vi "InterpretCLI.vi"(11 "Path":path) -> (1 "Strings":string[](array[string]), 2 "Layers":i32, 3 "Commands":T1(array[cluster]))   [LabVIEW 2012]
panel:
  out "MissedCommands":u16[](array[numeric])
  out "Command":u16
  out "TotalSize":i32
  out "Command":string
  out "Data":string
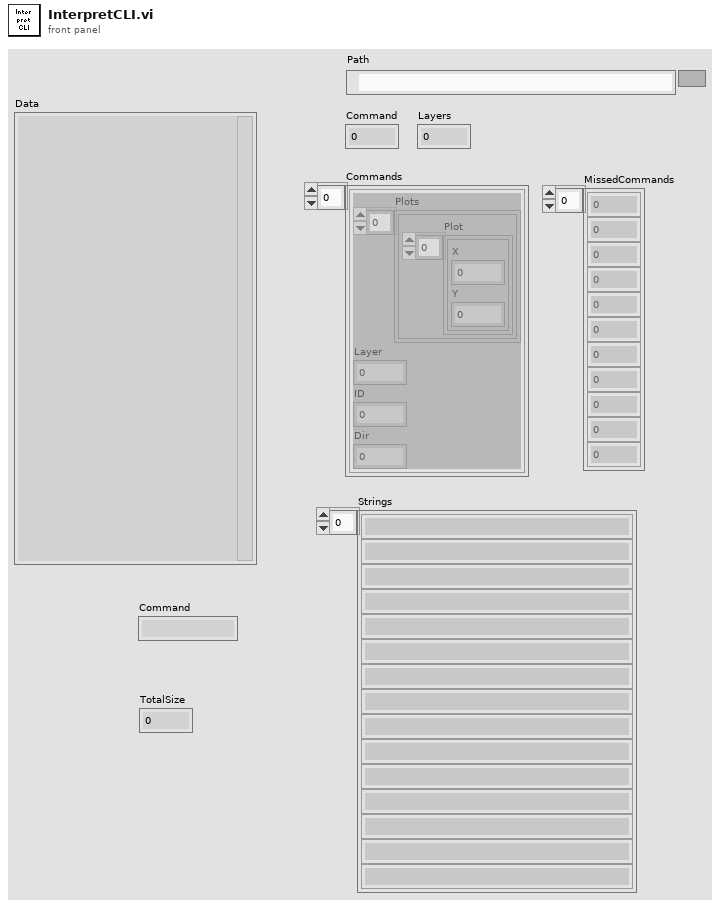
[diagram p1: front panel]
types:
  T1 = cluster{"Plots":cluster{"Plot":cluster{"X":dbl, "Y":dbl}[]}[], "Layer":dbl, "ID":dbl, "Dir":dbl}[]
  T2 = cluster{"Plots":cluster{"Plot":cluster{"X":dbl, "Y":dbl}[]}[], "Layer":dbl, "ID":dbl, "Dir":dbl}
  T3 = enum16{"big-endian, network order", "native, host order", "little-endian"}
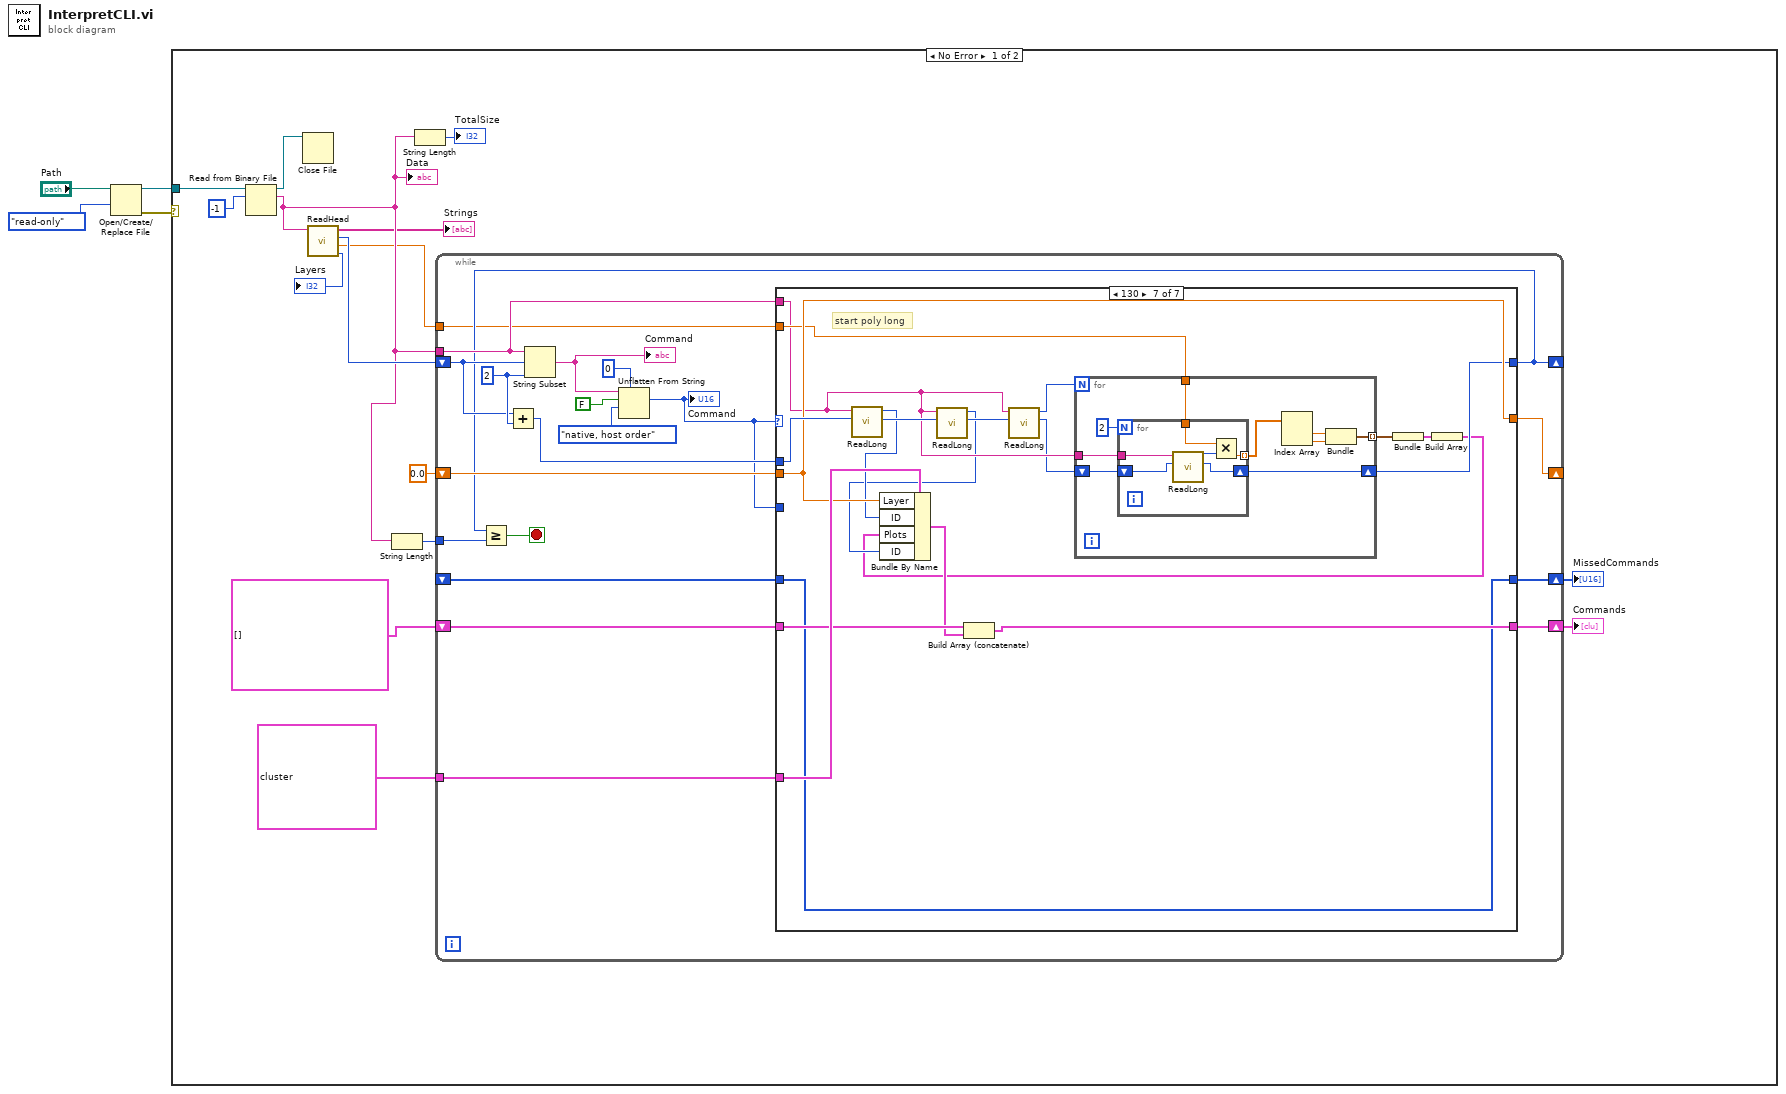
[diagram p0: block diagram]
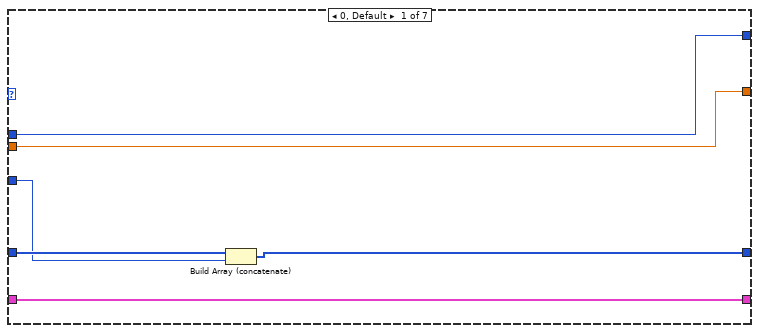
[diagram p2: hidden frame]
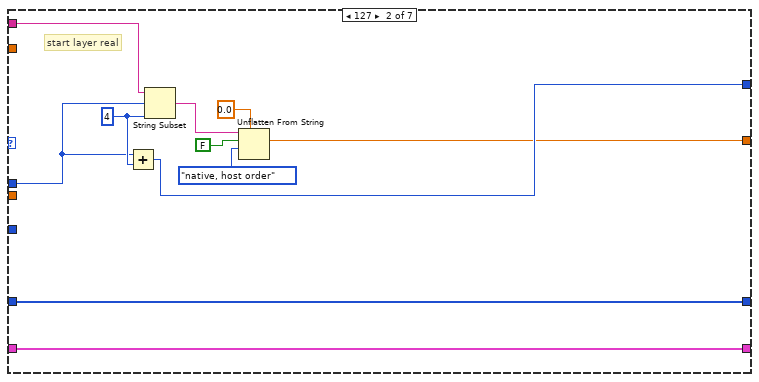
[diagram p3: hidden frame]
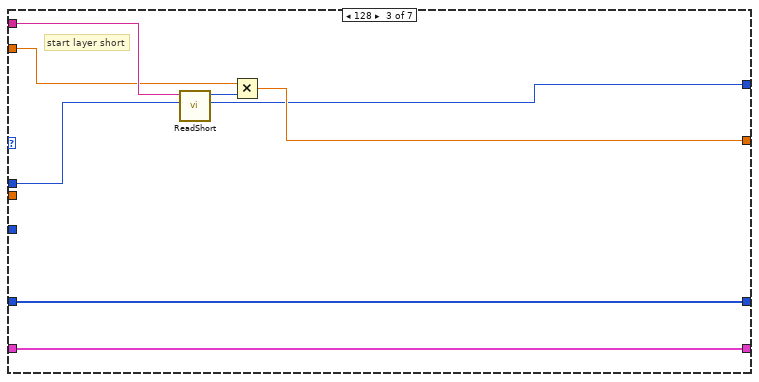
[diagram p4: hidden frame]
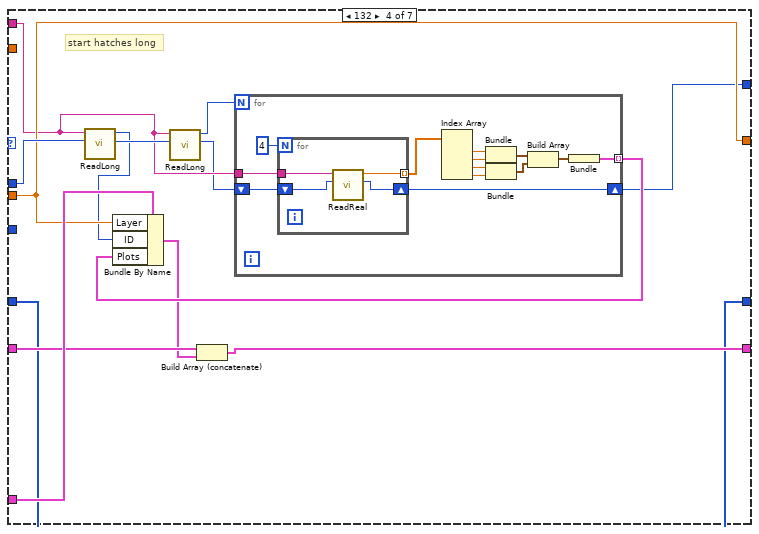
[diagram p5: hidden frame]
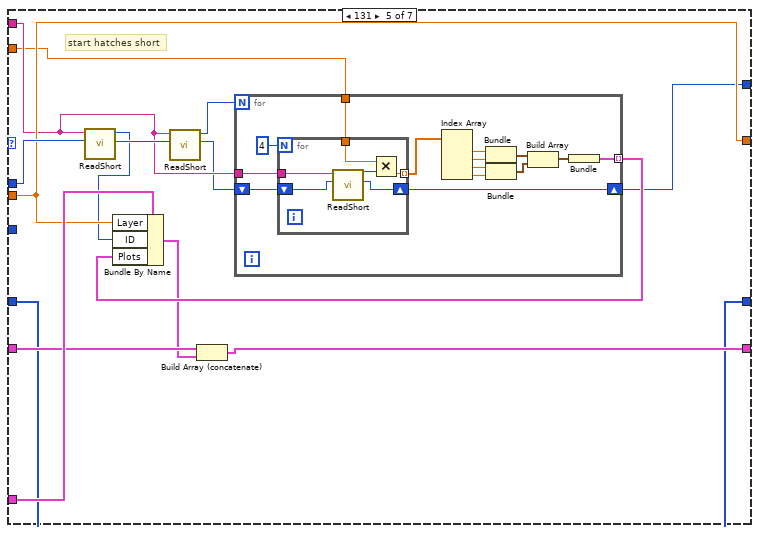
[diagram p6: hidden frame]
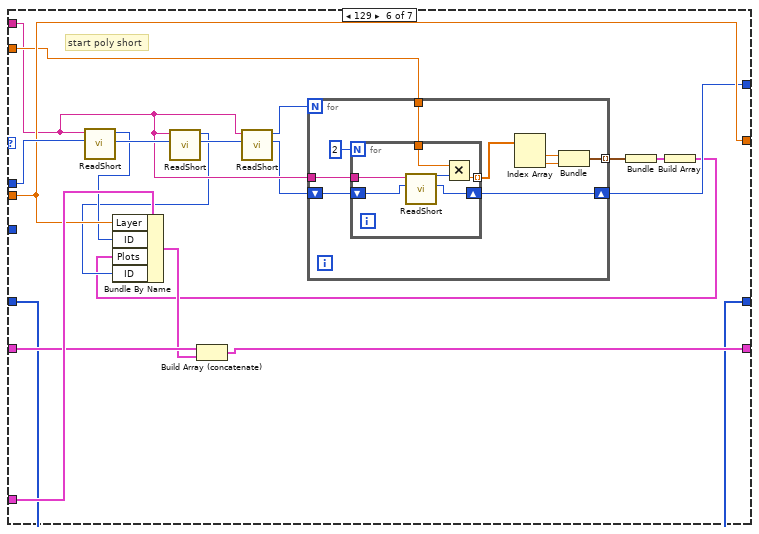
[diagram p7: hidden frame]
diagram:
  n1 = Open/Create/Replace File(file path (use dialog)="Path", access (0:read/write)=enum16{"read/write", "read-only", "write-only"}."read-only") -> (refnum out=w3:refnum<file>, error out=w1:errorcluster)  [unwired: 4 in, 1 out]
  n2 = case shown="No Error" w1 {
    tunnel: w3 -> [w19 _]
    frame No Error {
      n3 = Read from Binary File(10:-1 ("count (1)"), 11:w19) -> (2:w14:string, 3:w17:refnum<file>)  [unwired: 4 in, 2 out]
      "Data" <- w14
      n4 = Close File(refnum=w17) -> ()  [unwired: 1 in, 2 out]
      n5 = call "ReadHead.vi"("Data"=w14) -> ("Layers"=→"Layers":i32, "Units"=w6:dbl, "Off"=w15:u32, "Strings"=→"Strings":string[])  [unwired: 7 in]
      n6 = String Length(string=w14) -> (length=w12:i32)
      n7 = String Length(string=w14) -> (length=→"TotalSize":i32)
      n8 = while {
        tunnel: w14 -> [w33]
        shift-right: [w28] -> _
        shift-left: w15 -> [w29]
        shift-right: [w32] -> _
        shift-left: sgl 0.0 ("length (rest)") -> [w31]
        tunnel: w12 -> [w27]
        shift-right: [w25] -> w9
        shift-left: T1 [] -> [w24]
        tunnel: T2 {"Plots"=[{"Plot"=[{"X"=0.0, "Y"=0.0}, {"X"=1.0, "Y"=1.0}]}, {"Plot"=[{"X"=0.0, "Y"=1.0}, {"X"=1.0, "Y"=0.0}]}], "Layer"=0.0, "ID"=0.0, "Dir"=0.0} ("Command") -> [w26]
        shift-right: [w21] -> w7
        shift-left: _ -> [w22]
        tunnel: w6 -> [w20]
        stop <- w30 stop-if-true
        w35 = 2 ("length (rest)")
        n9 = Add(x=w29, y=w35) -> (x+y=w34:u32)
        n10 = String Subset(string=w33, offset (0)=w29, length (rest)=w35) -> (substring=w37:string)
        "Command" <- w37
        n11 = Unflatten From String(type=u16 0 ("length (rest)"), binary string=w37, data includes array or string size? (T)=FALSE, byte order (0:big-endian, network order)=T3."native, host order") -> (value=w23:u16)  [unwired: 1 in, 2 out]
        "Command" <- w23
        n12 = case shown="130" w23 {
          tunnel: w34 -> [w44 w50 w61 w78 w110 w149 w183]
          tunnel: w33 -> [_ w51 w62 w72 w104 w138 w172]
          tunnel: [w44 w49 w57 w69 w101 w144 w178] -> w28
          tunnel: [w45 w48 w58 w75 w107 w146 w180] -> w32
          tunnel: w31 -> [w45 _ _ w75 w107 w146 w180]
          tunnel: w26 -> [_ _ _ w76 w108 w147 w181]
          tunnel: [w43 w47 w64 w66 w98 w141 w175] -> w25
          tunnel: w24 -> [w43 w47 w64 w68 w100 w143 w177]
          tunnel: w23 -> [w41 _ _ _ _ _ _]
          tunnel: w22 -> [w42 w46 w63 w65 w97 w140 w174]
          tunnel: [w40 w46 w63 w65 w97 w140 w174] -> w21
          tunnel: w20 -> [_ _ w59 _ w96 w139 w173]
          frame 0, Default {
            n13 = Build Array (concatenate)(w42, w41) -> (w40:u16[])
          }
          frame 127 {
            w56 = 4 ("length (rest)")
            # "start layer real"
            n14 = Add(x=w50, y=w56) -> (x+y=w49:u32)
            n15 = String Subset(string=w51, offset (0)=w50, length (rest)=w56) -> (substring=w54:string)
            n16 = Unflatten From String(type=sgl 0.0 ("length (rest)"), binary string=w54, data includes array or string size? (T)=FALSE, byte order (0:big-endian, network order)=T3."native, host order") -> (value=w48:sgl)  [unwired: 1 in, 2 out]
          }
          frame 128 {
            # "start layer short"
            n17 = call "ReadShort.vi"("Offset"=w61, "Data"=w62) -> ("OffsetOut"=w57:u32, "Value"=w60:u16)  [unwired: 8 in]
            n18 = Multiply(x=w59, y=w60) -> (x*y=w58:dbl)
          }
          frame 132 {
            # "start hatches long"
            n19 = call "ReadLong.vi"("Offset"=w78, "Data"=w72) -> ("OffsetOut"=w77:u32, "Value"=w74:u32)  [unwired: 8 in]
            n20 = call "ReadLong.vi"("Offset"=w77, "Data"=w72) -> ("OffsetOut"=w71:u32, "Value"=w73:u32)  [unwired: 8 in]
            n21 = for {
              N: w73 -> [_]
              tunnel: w72 -> [w91]
              shift-right: [w88] -> w69
              shift-left: w71 -> [w89]
              tunnel: [w79] -> w70 mode=indexing
              n22 = for {
                N: 4 -> [_]
                tunnel: w91 -> [w95]
                shift-right: [w93] -> w88
                shift-left: w89 -> [w94]
                tunnel: [w92] -> w87 mode=indexing
                n23 = call "ReadReal.vi"("Offset"=w94, "Data"=w95) -> ("OffsetOut"=w93:u32, "Value"=w92:sgl)  [unwired: 8 in]
              }
              n24 = Index Array(array=w87) -> (element #1=w86:sgl, element #2=w85:sgl, element #3=w84:sgl, element #4=w83:sgl)  [unwired: 4 in]
              n25 = Bundle("Value"=w86, "Value"=w85) -> (w82:cluster{"Value":sgl, "Value":sgl})  [unwired: 1 in]
              n26 = Bundle("Value"=w84, "Value"=w83) -> (w81:cluster{"Value":sgl, "Value":sgl})  [unwired: 1 in]
              n27 = Build Array(w82, w81) -> (w80:cluster{"Value":sgl, "Value":sgl}[])
              n28 = Bundle(w80) -> (w79:cluster{cluster{"Value":sgl, "Value":sgl}[]})  [unwired: 1 in]
            }
            n29 = Bundle By Name(cluster=w76, "Layer"=w75, "ID"=w74, "Plots"=w70) -> (w67:T2)
            n30 = Build Array (concatenate)(w68, w67) -> (w66:T1)
          }
          frame 131 {
            # "start hatches short"
            n31 = call "ReadShort.vi"("Offset"=w110, "Data"=w104) -> ("OffsetOut"=w109:u32, "Value"=w106:u16)  [unwired: 8 in]
            n32 = call "ReadShort.vi"("Offset"=w109, "Data"=w104) -> ("OffsetOut"=w103:u32, "Value"=w105:u16)  [unwired: 8 in]
            n33 = for {
              N: w105 -> [_]
              tunnel: w104 -> [w124]
              shift-right: [w121] -> w101
              shift-left: w103 -> [w122]
              tunnel: [w112] -> w102 mode=indexing
              tunnel: w96 -> [w111]
              n34 = for {
                N: 4 -> [_]
                tunnel: w124 -> [w130]
                shift-right: [w128] -> w121
                shift-left: w122 -> [w129]
                tunnel: [w126] -> w120 mode=indexing
                tunnel: w111 -> [w125]
                n35 = call "ReadShort.vi"("Offset"=w129, "Data"=w130) -> ("OffsetOut"=w128:u32, "Value"=w127:u16)  [unwired: 8 in]
                n36 = Multiply(x=w125, y=w127) -> (x*y=w126:dbl)
              }
              n37 = Index Array(array=w120) -> (element #1=w119:dbl, element #2=w118:dbl, element #3=w117:dbl, element #4=w116:dbl)  [unwired: 4 in]
              n38 = Bundle(w119, w118) -> (w115:cluster{dbl, dbl})  [unwired: 1 in]
              n39 = Bundle(w117, w116) -> (w114:cluster{dbl, dbl})  [unwired: 1 in]
              n40 = Build Array(w115, w114) -> (w113:cluster{dbl, dbl}[])
              n41 = Bundle(w113) -> (w112:cluster{cluster{dbl, dbl}[]})  [unwired: 1 in]
            }
            n42 = Bundle By Name(cluster=w108, "Layer"=w107, "ID"=w106, "Plots"=w102) -> (w99:T2)
            n43 = Build Array (concatenate)(w100, w99) -> (w98:T1)
          }
          frame 129 {
            # "start poly short"
            n44 = call "ReadShort.vi"("Offset"=w149, "Data"=w138) -> ("OffsetOut"=w148:u32, "Value"=w145:u16)  [unwired: 8 in]
            n45 = call "ReadShort.vi"("Offset"=w148, "Data"=w138) -> ("OffsetOut"=w137:u32, "Value"=w134:u16)  [unwired: 8 in]
            n46 = call "ReadShort.vi"("Offset"=w137, "Data"=w138) -> ("OffsetOut"=w136:u32, "Value"=w135:u16)  [unwired: 8 in]
            n47 = for {
              N: w135 -> [_]
              tunnel: w138 -> [w158]
              shift-right: [w155] -> w144
              shift-left: w136 -> [w156]
              tunnel: [w150] -> w133 mode=indexing
              tunnel: w139 -> [w151]
              n48 = for {
                N: 2 -> [_]
                tunnel: w158 -> [w164]
                shift-right: [w162] -> w155
                shift-left: w156 -> [w163]
                tunnel: [w160] -> w154 mode=indexing
                tunnel: w151 -> [w159]
                n49 = call "ReadShort.vi"("Offset"=w163, "Data"=w164) -> ("OffsetOut"=w162:u32, "Value"=w161:u16)  [unwired: 8 in]
                n50 = Multiply(x=w159, y=w161) -> (x*y=w160:dbl)
              }
              n51 = Index Array(array=w154) -> (element #1=w153:dbl, element #2=w152:dbl)  [unwired: 2 in]
              n52 = Bundle(w153, w152) -> (w150:cluster{dbl, dbl})  [unwired: 1 in]
            }
            n53 = Bundle(w133) -> (w132:cluster{cluster{dbl, dbl}[]})  [unwired: 1 in]
            n54 = Build Array(w132) -> (w131:cluster{cluster{dbl, dbl}[]}[])
            n55 = Bundle By Name(cluster=w147, "Layer"=w146, "ID"=w145, "Plots"=w131, "ID"=w134) -> (w142:T2)
            n56 = Build Array (concatenate)(w143, w142) -> (w141:T1)
          }
          frame 130 {
            # "start poly long"
            n57 = call "ReadLong.vi"("Offset"=w183, "Data"=w172) -> ("OffsetOut"=w182:u32, "Value"=w179:u32)  [unwired: 8 in]
            n58 = call "ReadLong.vi"("Offset"=w182, "Data"=w172) -> ("OffsetOut"=w171:u32, "Value"=w168:u32)  [unwired: 8 in]
            n59 = call "ReadLong.vi"("Offset"=w171, "Data"=w172) -> ("OffsetOut"=w170:u32, "Value"=w169:u32)  [unwired: 8 in]
            n60 = for {
              N: w169 -> [_]
              tunnel: w172 -> [w192]
              shift-right: [w189] -> w178
              shift-left: w170 -> [w190]
              tunnel: [w184] -> w167 mode=indexing
              tunnel: w173 -> [w185]
              n61 = for {
                N: 2 -> [_]
                tunnel: w192 -> [w198]
                shift-right: [w196] -> w189
                shift-left: w190 -> [w197]
                tunnel: [w194] -> w188 mode=indexing
                tunnel: w185 -> [w193]
                n62 = call "ReadLong.vi"("Offset"=w197, "Data"=w198) -> ("OffsetOut"=w196:u32, "Value"=w195:u32)  [unwired: 8 in]
                n63 = Multiply(x=w193, y=w195) -> (x*y=w194:dbl)
              }
              n64 = Index Array(array=w188) -> (element #1=w187:dbl, element #2=w186:dbl)  [unwired: 2 in]
              n65 = Bundle(w187, w186) -> (w184:cluster{dbl, dbl})  [unwired: 1 in]
            }
            n66 = Bundle(w167) -> (w166:cluster{cluster{dbl, dbl}[]})  [unwired: 1 in]
            n67 = Build Array(w166) -> (w165:cluster{cluster{dbl, dbl}[]}[])
            n68 = Bundle By Name(cluster=w181, "Layer"=w180, "ID"=w179, "Plots"=w165, "ID"=w168) -> (w176:T2)
            n69 = Build Array (concatenate)(w177, w176) -> (w175:T1)
          }
        }
        n70 = Greater Or Equal?(x=w28, y=w27) -> (x >= y?=w30:bool)
      }
      "Commands" <- w9
      "MissedCommands" <- w7
    }
    frame Error {
    }
  }
